vi "Get SMO Database Paths.vi"(5 "getAll Cluster":variant, 7 "Paths":string="llab_038:d000(TEST_TABLE--Temperature(Kelvin))\nllab_038:d002(TEST_TABLE--voltage 2(volts))\nllab_038:b000(TEST_TABLE--ON?())\nllab_038:v001(TEST_TABLE--sample())", 8 "error in (no error)":errorcluster, 11 "Inst.Transport in":refnum<class "Inst.Transport.lvclass">) -> (0 "error out":errorcluster, 2 "Paths":string, 3 "Inst.Transport out":refnum<class "Inst.Transport.lvclass">)   [LabVIEW 2019, in "Inst.Transport.lvclass"]
uses:
  Inst.Transport.lvclass
  Typedefs/Inst.Transport.getAll--Cluster.ctl
  <userlib>/LevyLab/Instrument Framework/Instrument Types/SCPI/Instrument.SCPI.lvclass
  <userlib>/LevyLab/LV-Data/LV-Data.PG/LV-Data.PGSQL.lvclass
  <userlib>/LevyLab/LV-Data/LV-Data.PG/API/Write Variable (one-row).vi
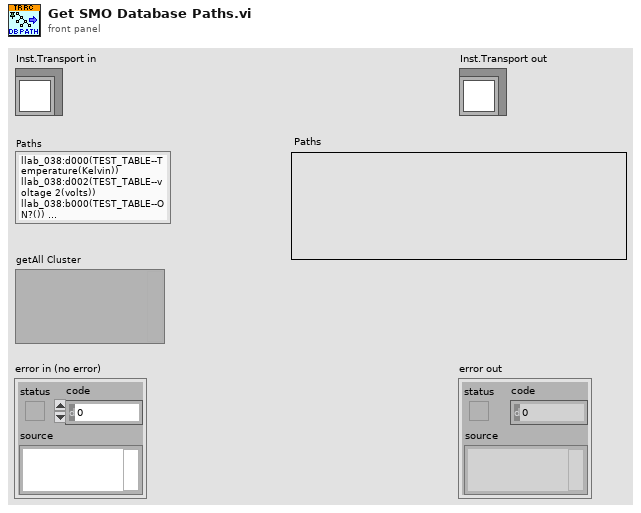
[diagram p1: front panel]
types:
  T1 = typedef "Inst.Transport.lvclass/Inst.Transport.getAll--Cluster.ctl" = cluster{"data":variant}
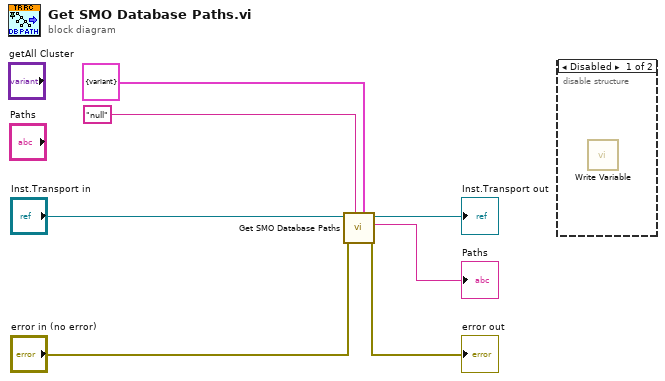
[diagram p0: block diagram]
diagram:
  n1 = call-parent "Get SMO Database Paths.vi"("getAll Cluster"=T1 {"data"=variant(string "")} ("getAll"), "Default Paths"="null" ("Paths"), "error in (no error)"="error in (no error)", "Instrument in"="Inst.Transport in") -> ("error out"=→"error out":errorcluster, "Paths"=→"Paths":string, "Instrument out"=→"Inst.Transport out":refnum<class "Inst.Transport.lvclass">)  [unwired: 5 in]
  n2 = disable-structure shown="Disabled" {
    frame Disabled {
      n3 = call-poly <userlib>:"Write Variable.vi"() -> ()  [unwired: 8 in, 4 out]
    }
    frame Enabled {
    }
  }
